vi "Select ID By Name.vi"(7 "Name":string, 8 "Error In":errorcluster, 9 "Column (id)":string="id", 10 "Table":string, 11 "connection reference":T1) -> (0 "Error Out":errorcluster, 1 "ID":i32, 3 "dup connection reference":T1)   [LabVIEW 2016, in "DB-Configuration.lvlib"]
doc: "select ID from Table where name = 'Name';"
uses:
  DB-Configuration.lvlib
  <vilib>/addons/database/Connection.llb/Conn ObjectReference.ctl
  <vilib>/addons/database/_DB Variant To Data/Database Variant To Data.xnode
  <vilib>/addons/database/NI_Database_API.lvlib
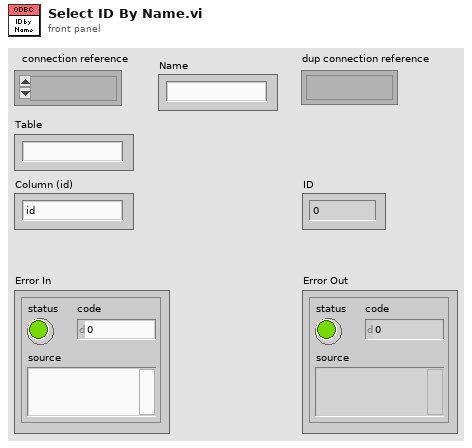
[diagram p1: front panel]
types:
  T1 = typedef "NI_Database_API.lvlib/Conn ObjectReference.ctl" = refnum<k1>
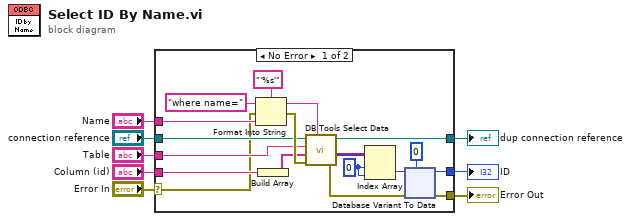
[diagram p0: block diagram]
diagram:
  n1 = case shown="No Error" "Error In" {
    selector: "Error In" -> [w9 w59]
    tunnel: "connection reference" -> [w19 w60]
    tunnel: [w18 w60] -> w7
    tunnel: "Column (id)" -> [w15 _]
    tunnel: "Name" -> [w13 _]
    tunnel: [w12 _] -> w4
    tunnel: "Table" -> [w11 _]
    tunnel: [w10 w59] -> w2
    frame No Error {
      w21 = 0 ("index (row)")
      n2 = Format Into String(format string="'%s'", initial string="where name=", error in=w9, w13) -> (resulting string=w26:string, error out=w25:errorcluster)
      n3 = Build Array(w15) -> (w14:string[])
      n4 = call <vilib>:"DB Tools Select Data.vi"("condition"=w26, "error in (no error)"=w25, "columns"=w14, "table"=w11, "connection reference"=w19) -> ("error out"=w17:errorcluster, "data"=w23:variant[][], "connection reference out"=w18:T1)  [unwired: 1 in]
      n5 = Index Array(array=w23, index (row)=w21, index (col)=w21) -> (element=w22:variant)
      n6 = xnode "Database Variant To Data"("database variant"=w22, "error in (no error)"=w17, "type"=0) -> ("data"=w12:i32, "error out"=w10:errorcluster)
    }
    frame Error {
    }
  }
  "dup connection reference" <- w7
  "ID" <- w4
  "Error Out" <- w2
